vi "Write.vi"(8 "Error In":errorcluster, 10 "Content":string, 11 "Writer In":refnum<class "String.lvclass">) -> (0 "Error Out":errorcluster, 3 "Writer Out":refnum<class "String.lvclass">)   [LabVIEW 2018, in "Toolkit.lvlib" / "Writers.lvlib" / "String.lvclass"]
uses:
  String.lvclass
  String.lvclass/String.ctl
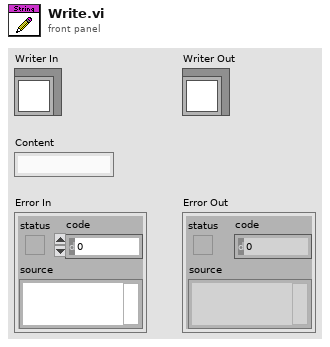
[diagram p1: front panel]
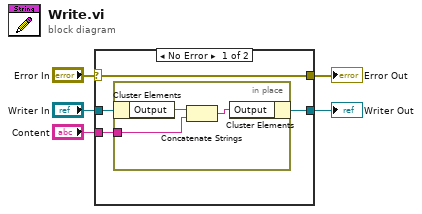
[diagram p0: block diagram]
diagram:
  n1 = case shown="No Error" "Error In" {
    selector: "Error In" -> [w7 w13]
    tunnel: "Writer In" -> [w9 w14]
    tunnel: [w8 w14] -> w3
    tunnel: [w7 w13] -> w2
    tunnel: "Content" -> [w6 _]
    frame No Error {
      n2 = in-place {
        in-place-border: w6 -> [w10]
        n3 = in-place-cluster #1(w9) -> ("Output"=w12:string)
        n4 = Concatenate Strings(w12, w10) -> (w11:string)
        n5 = in-place-cluster #1("Output"=w11) -> (w8:refnum<class "String.lvclass">)
      }
    }
    frame Error {
    }
  }
  "Error Out" <- w2
  "Writer Out" <- w3
